vi "getRef.vi"(8 "Error out":errorcluster caption="error in", 10 "Name":string, 11 "Gen ref in":refnum<vi>) -> (0 "Error out":errorcluster caption="error out", 2 "Cousins":string, 3 "Gen ref out":refnum<vi>)   [LabVIEW 2017]
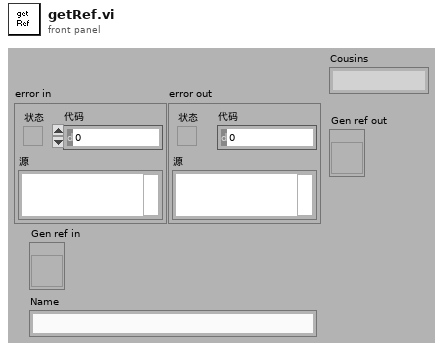
[diagram p1: front panel]
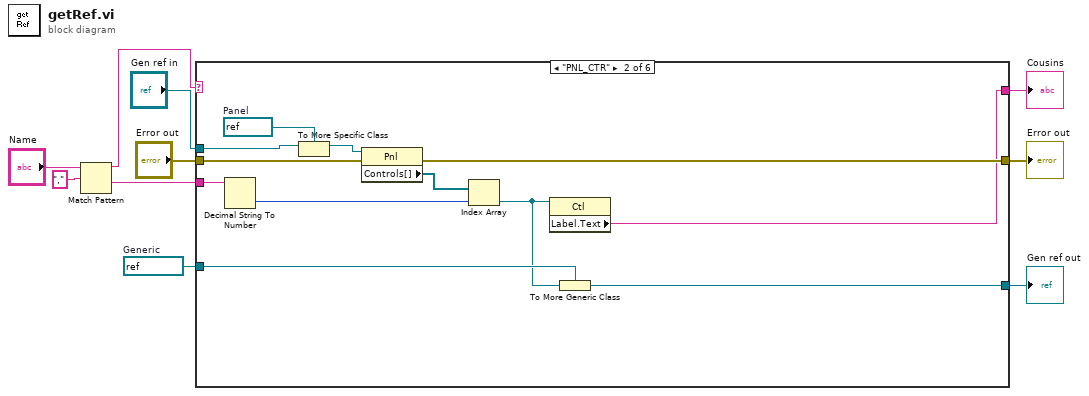
[diagram p0: block diagram]
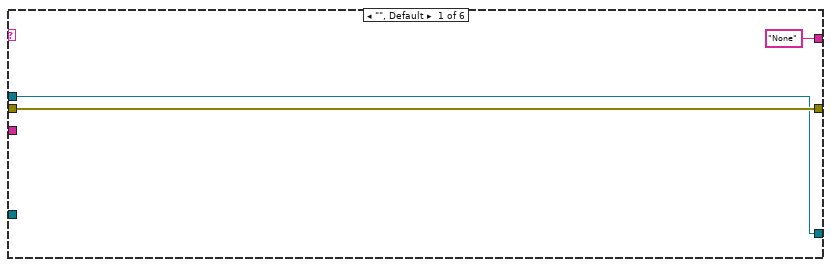
[diagram p2: hidden frame]
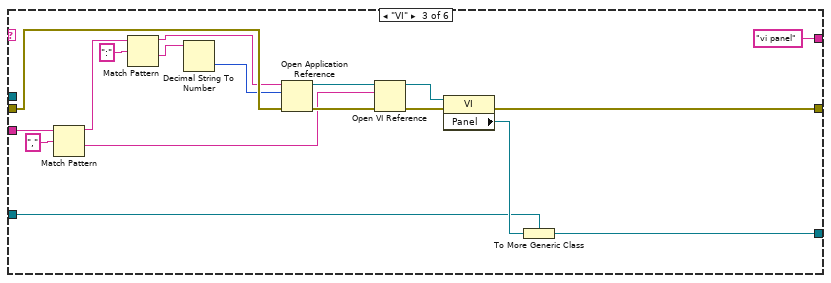
[diagram p3: hidden frame]
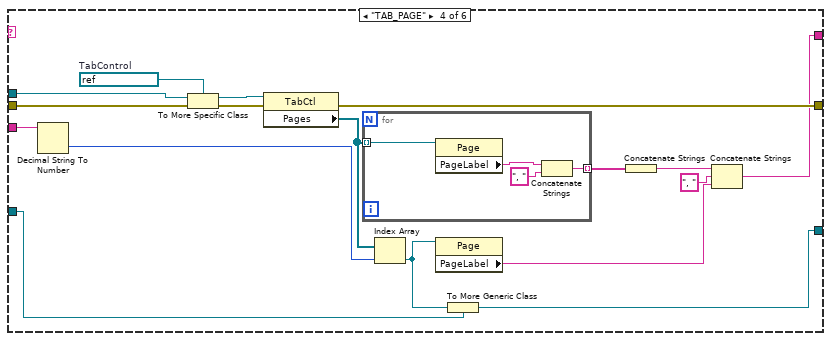
[diagram p4: hidden frame]
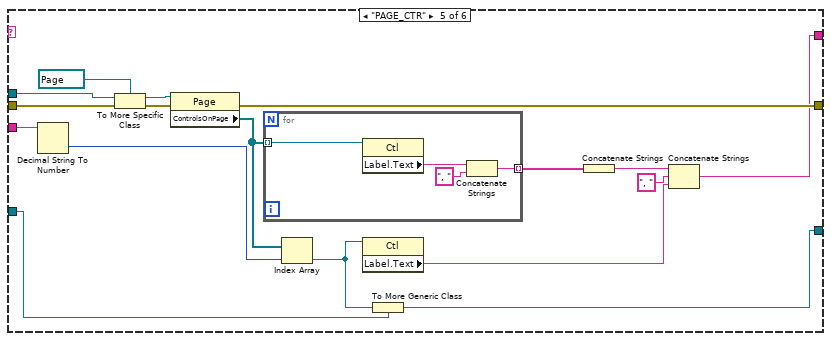
[diagram p5: hidden frame]
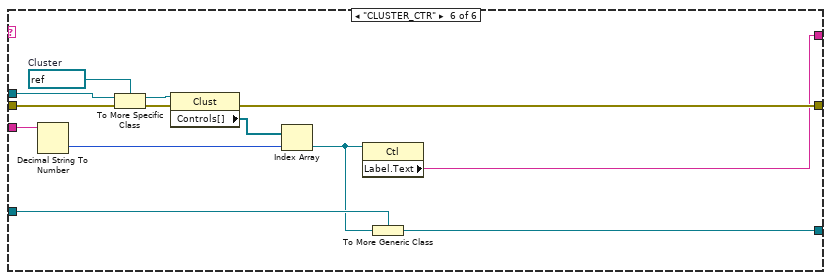
[diagram p6: hidden frame]
diagram:
  w3 = refnum<vi> refnum  # Generic
  n1 = Match Pattern(string="Name", regular expression="," ("正则表达式")) -> (before substring=w6:string, after substring=w5:string)  [unwired: 3 out]
  n2 = case shown="\"PNL_CTR\"" w6 {
    tunnel: "Error out" -> [w13 w20 w39 w57 w75 w90]
    tunnel: [w13 w17 w28 w53 w73 w89] -> w9
    tunnel: w5 -> [_ w19 w38 w56 w77 w91]
    tunnel: [w12 w24 w31 w55 w78 w88] -> w2
    tunnel: "Gen ref in" -> [w12 w23 _ w58 w80 w94]
    tunnel: w3 -> [_ w16 w27 w52 w72 w92]
    tunnel: ["None" ("Label.Text") w14 "vi panel" ("Label.Text") w46 w67 w86] -> w1
    frame "", Default {
    }
    frame "PNL_CTR" {
      w22 = refnum<vi> refnum  # Panel
      n3 = Decimal String To Number(string=w19) -> (number=w18:i32)  [unwired: 3 out]
      n4 = To More Specific Class(target class=w22, reference=w23) -> (specific class reference=w21:refnum<vi>)  [unwired: 1 in, 1 out]
      n5 = property class="Pnl"(reference=w21, error in=w20) -> (error out=w17:errorcluster, "Controls[]"=w25:refnum<vi>[])  [unwired: 1 out]
      n6 = Index Array(array=w25, index=w18) -> (element=w15:refnum<vi>)
      n7 = property class="Ctl"(reference=w15) -> ("Label.Text"=w14:string)  [unwired: 1 in, 2 out]
      n8 = To More Generic Class(target class=w16, reference=w15) -> (generic class reference=w24:refnum<vi>)
    }
    frame "VI" {
      n9 = Match Pattern(string=w38, regular expression="," ("正则表达式")) -> (before substring=w35:string, after substring=w33:string)  [unwired: 3 out]
      n10 = Match Pattern(string=w35, regular expression=":" ("正则表达式")) -> (before substring=w34:string, after substring=w30:string)  [unwired: 3 out]
      n11 = Decimal String To Number(string=w30) -> (number=w29:i32)  [unwired: 3 out]
      n12 = Open Application Reference(8:w39, 10:w29, 11:w34) -> (0:w41:errorcluster, 3:w42:refnum<vi>)  [unwired: 1 out]
      n13 = Open VI Reference(application reference (local)=w42, vi path=w33, error in (no error)=w41) -> (vi reference=w43:refnum<vi>, error out=w40:errorcluster)  [unwired: 3 out]
      n14 = property class="VI"(reference=w43, error in=w40) -> (error out=w28:errorcluster, "Panel"=w32:refnum<vi>)  [unwired: 1 out]
      n15 = To More Generic Class(target class=w27, reference=w32) -> (generic class reference=w31:refnum<vi>)
    }
    frame "TAB_PAGE" {
      w59 = refnum<vi> refnum  # TabControl
      n16 = Decimal String To Number(string=w56) -> (number=w54:i32)  [unwired: 3 out]
      n17 = To More Specific Class(target class=w59, reference=w58, error in=w57) -> (specific class reference=w50:refnum<vi>, error out=w60:errorcluster)
      n18 = property class="TabCtl"(reference=w50, error in=w60) -> (error out=w53:errorcluster, "Pages"=w49:refnum<vi>[])  [unwired: 1 out]
      n19 = for {
        tunnel: w49 -> [w64] mode=indexing
        tunnel: [w62] -> w48 mode=indexing
        n20 = property class="Page"(reference=w64) -> ("PageLabel"=w63:string)  [unwired: 1 in, 2 out]
        n21 = Concatenate Strings(w63, ", " ("string")) -> (w62:string)
      }
      n22 = Index Array(array=w49, index=w54) -> (element=w51:refnum<vi>)
      n23 = property class="Page"(reference=w51) -> ("PageLabel"=w45:string)  [unwired: 1 in, 2 out]
      n24 = To More Generic Class(target class=w52, reference=w51) -> (generic class reference=w55:refnum<vi>)
      n25 = Concatenate Strings(w48) -> (w47:string)
      n26 = Concatenate Strings(w47, ", " ("string"), w45) -> (w46:string)
    }
    frame "PAGE_CTR" {
      n27 = Decimal String To Number(string=w77) -> (number=w76:i32)  [unwired: 3 out]
      n28 = To More Specific Class(target class=refnum<vi> refnum ("元素"), reference=w80, error in=w75) -> (specific class reference=w79:refnum<vi>, error out=w81:errorcluster)
      n29 = property class="Page"(reference=w79, error in=w81) -> (error out=w73:errorcluster, "ControlsOnPage"=w70:refnum<vi>[])  [unwired: 1 out]
      n30 = for {
        tunnel: w70 -> [w85] mode=indexing
        tunnel: [w82] -> w69 mode=indexing
        n31 = property class="Ctl"(reference=w85) -> ("Label.Text"=w83:string)  [unwired: 1 in, 2 out]
        n32 = Concatenate Strings(w83, ", " ("string")) -> (w82:string)
      }
      n33 = Index Array(array=w70, index=w76) -> (element=w71:refnum<vi>)
      n34 = property class="Ctl"(reference=w71) -> ("Label.Text"=w65:string)  [unwired: 1 in, 2 out]
      n35 = To More Generic Class(target class=w72, reference=w71) -> (generic class reference=w78:refnum<vi>)
      n36 = Concatenate Strings(w69) -> (w68:string)
      n37 = Concatenate Strings(w68, ", " ("string"), w65) -> (w67:string)
    }
    frame "CLUSTER_CTR" {
      w93 = refnum<vi> refnum  # Cluster
      n38 = Decimal String To Number(string=w91) -> (number=w95:i32)  [unwired: 3 out]
      n39 = To More Specific Class(target class=w93, reference=w94, error in=w90) -> (specific class reference=w96:refnum<vi>, error out=w97:errorcluster)
      n40 = property class="Clust"(reference=w96, error in=w97) -> (error out=w89:errorcluster, "Controls[]"=w98:refnum<vi>[])  [unwired: 1 out]
      n41 = Index Array(array=w98, index=w95) -> (element=w87:refnum<vi>)
      n42 = property class="Ctl"(reference=w87) -> ("Label.Text"=w86:string)  [unwired: 1 in, 2 out]
      n43 = To More Generic Class(target class=w92, reference=w87) -> (generic class reference=w88:refnum<vi>)
    }
  }
  "Error out" <- w9
  "Gen ref out" <- w2
  "Cousins" <- w1
